vi "testslide.vi"   [LabVIEW 2019]
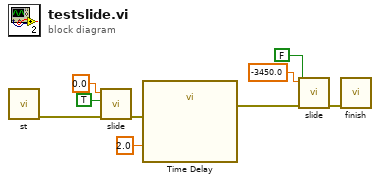
[diagram p0: block diagram]
diagram:
  n1 = call "st.vi"() -> ("Error/Flow Out"=w9:errorcluster)  [unwired: 11 in]
  n2 = call "slide.vi"("error in (no error)"=w9, "Reset Counter"=TRUE, "Numeric"=0.0) -> ("error out"=w5:errorcluster)  [unwired: 6 in, 2 out]
  n3 = call "Time Delay"("error in (no error)"=w5, "Delay Time (s)"=2.0) -> ("error out"=w4:errorcluster)  [unwired: 9 in]
  n4 = call "slide.vi"("error in (no error)"=w4, "Reset Counter"=FALSE, "Numeric"=-3450.0) -> ("error out"=w8:errorcluster)  [unwired: 6 in, 2 out]
  n5 = call "finish.vi"("Error/Flow In"=w8) -> ()  [unwired: 11 in]
